vi "Send Async Loop Error.vi"(8 "error in (no error)":errorcluster, 11 "Measurement UI Queue":refnum<queue>) -> (0 "error out":errorcluster)   [LabVIEW 2025, in "I2C Bus Monitor UI.lvlib"]
uses:
  I2C Bus Monitor UI.lvlib
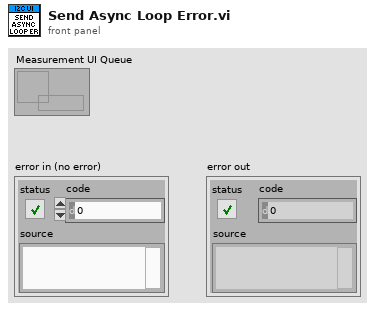
[diagram p1: front panel]
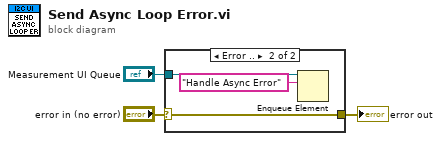
[diagram p0: block diagram]
diagram:
  n1 = case shown="Error .." "error in (no error)" {
    selector: "error in (no error)" -> [w4 w5]
    tunnel: "Measurement UI Queue" -> [_ w7]
    tunnel: [w4 w5] -> w2
    frame No Error {
    }
    frame Error {
      n2 = Enqueue Element(queue=w7, element="Handle Async Error") -> ()  [unwired: 2 in, 3 out]
    }
  }
  "error out" <- w2
